vi "Subroutine Example.vi"() -> ()   [LabVIEW 2019]
uses:
  <vilib>/gpm_packages/@cs/test-executive/Source/Test Executive/TestExecutive/Test Executive.lvclass
  C:/Program Files/National Instruments/LabVIEW 2019/vi.lib/gpm_packages/@cs/test-executive/Source/Test Executive/ITestExecutive/ITest Executive.lvclass
  <vilib>/gpm_packages/@cs/persistence/source/XML/XML.lvclass
  C:/Program Files/National Instruments/LabVIEW 2019/vi.lib/gpm_packages/@cs/persistence/source/IPersist/IPersist.lvclass
  <vilib>/gpm_packages/@cs/test-executive/Source/Test Executive/Executioner/Executioner.lvclass
  <vilib>/gpm_packages/@cs/test-executive/Source/Test Executive/TestExecutive Ref/TestExecutive Ref.lvclass
  907dcd56-9374-434c-9b61-223c76acbea6.vi
  b311528a-8885-46dc-880b-1248f53f849d.vi
  <vilib>/gpm_packages/@cs/run-time-assertions/Source/Assert Equal/Assert Equal.lvclass
  cdae3e82-8768-4ad8-b607-63d253822acd.vi
  70d01af1-a21d-4a89-960c-204e12f52ec9.vi
  fcedef66-c37f-4fec-9b65-1c54ba2e8624.vi
  f2235a25-2eab-467c-a315-b32e95189d54.vi
  <vilib>/gpm_packages/@cs/test-executive/Source/Sandbox/While Loop Stop Example/Mock Executioner/Mock Executioner.lvclass
  65bccb3a-65fa-47ab-80ee-1967ce04f6c9.vi
  06bca68b-79a8-4024-9cd4-aed976a9ea7c.vi
  43d0685a-3af2-457a-b80b-c7e9f70f9eef.vi
  a6ff4ce3-d06d-4066-9c6d-186ba633a42e.vi
  C:/Program Files/National Instruments/LabVIEW 2019/vi.lib/gpm_packages/@cs/run-time-assertions/Source/Assert/Assert.lvclass
panel:
  out "Active Unique ID out":string
  out "Value":i32
  in  "Subroutine Test Exec":string(tree)
  in  "stop":bool
  in  "Saved Test Exec":string(tree)
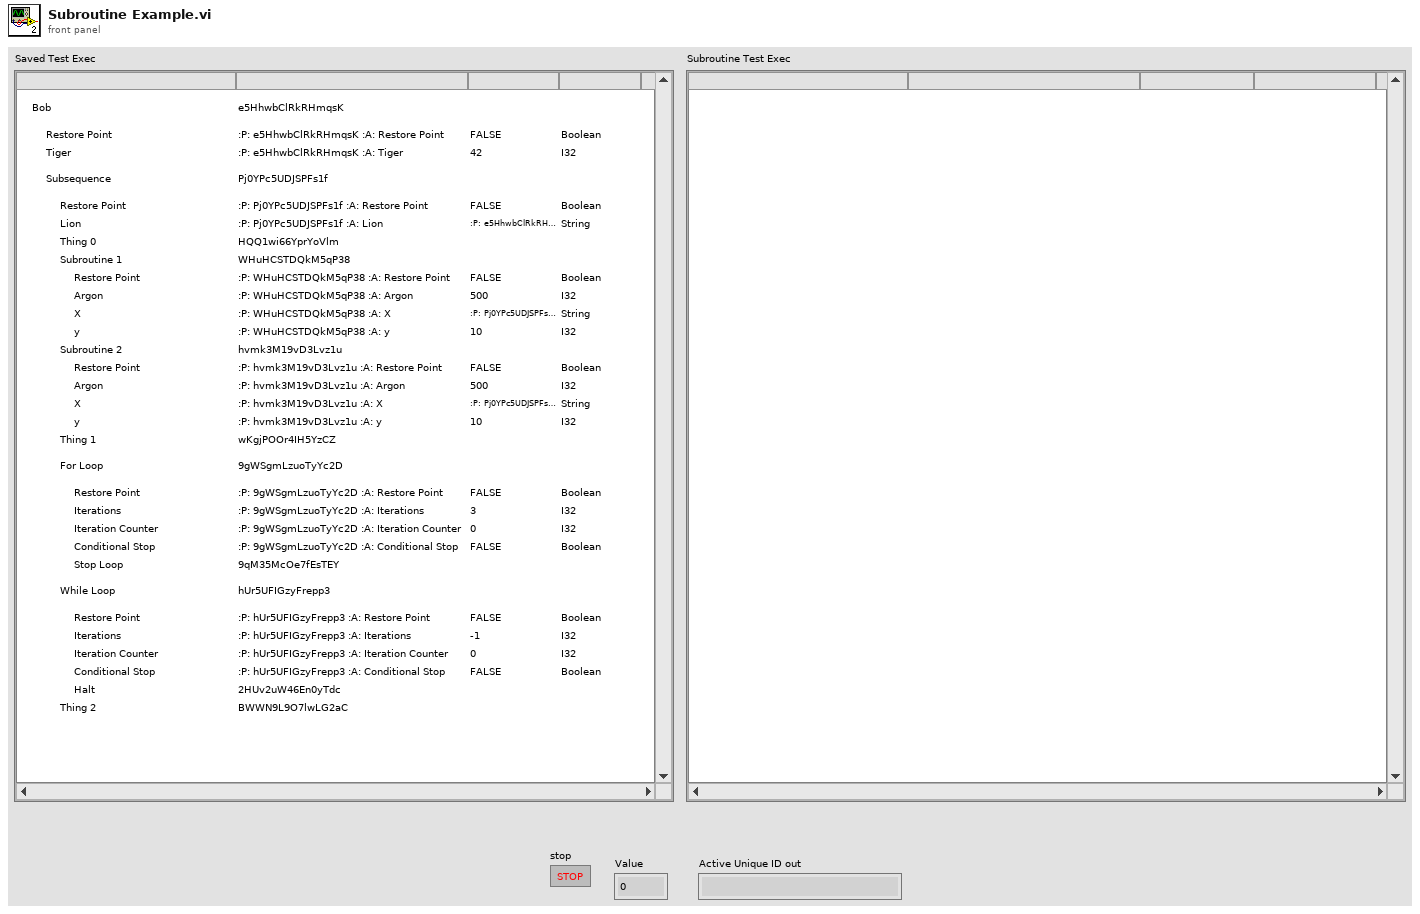
[diagram p1: front panel]
types:
  T1 = cluster{"Left Cell String":string, "Child Text":string[], "Child Tag":string, "Item Indent":i32, "Child Only?":bool, "Glyph Index":i32}[]
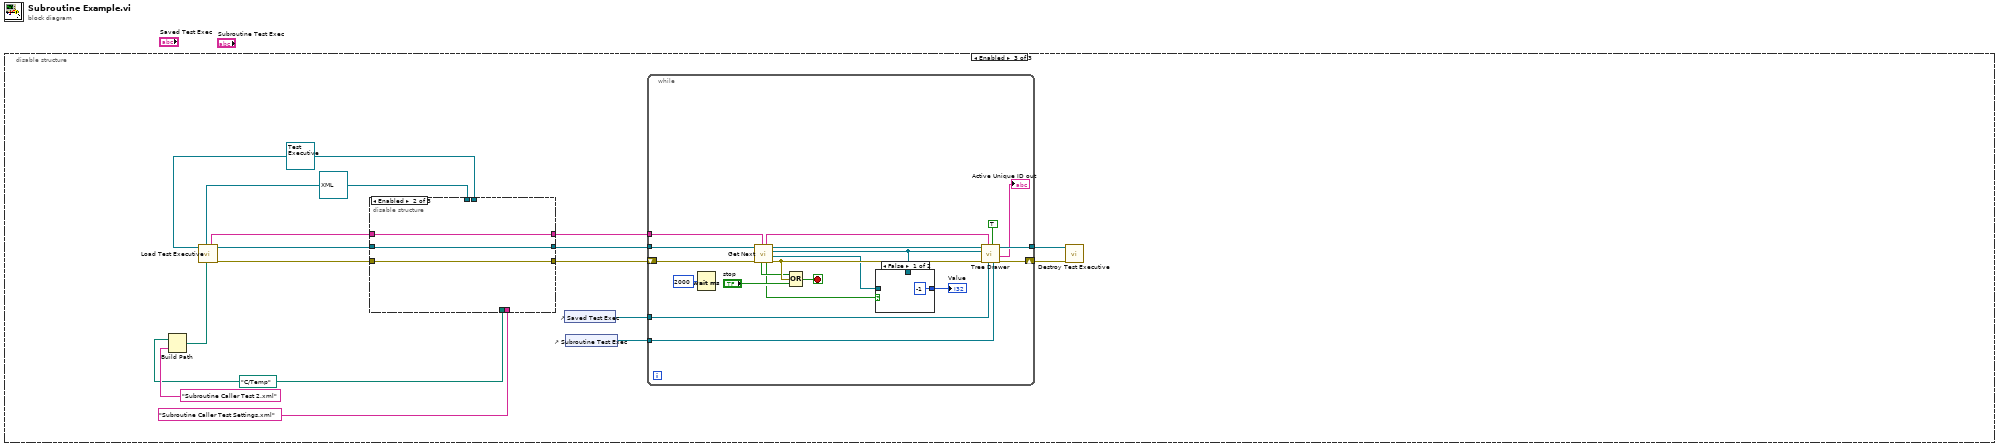
[diagram p0: block diagram]
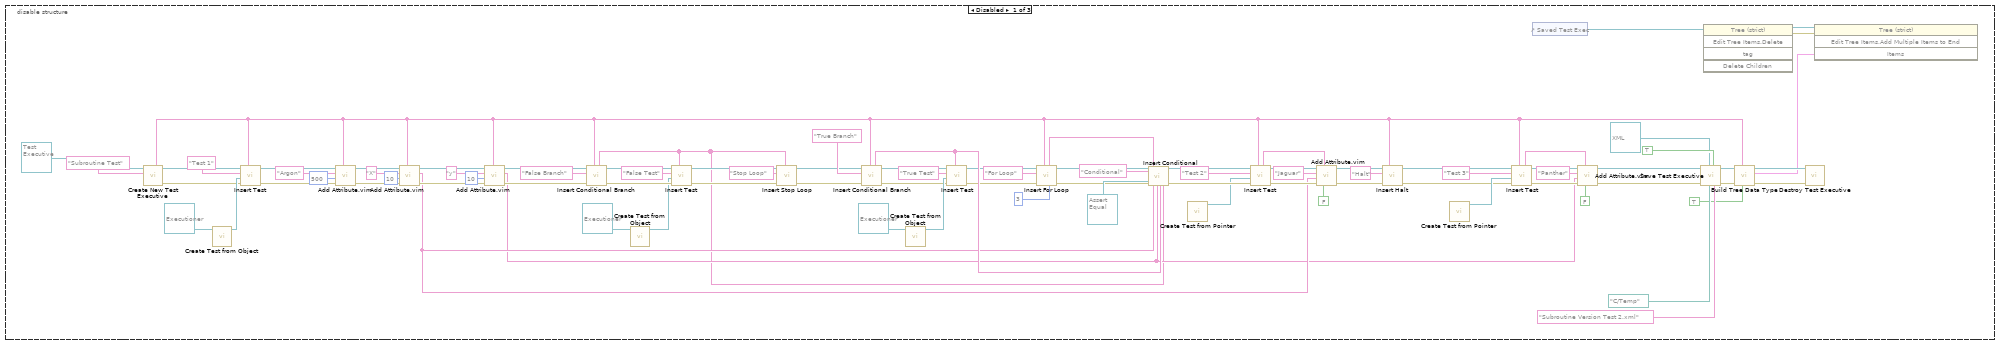
[diagram p2: hidden frame]
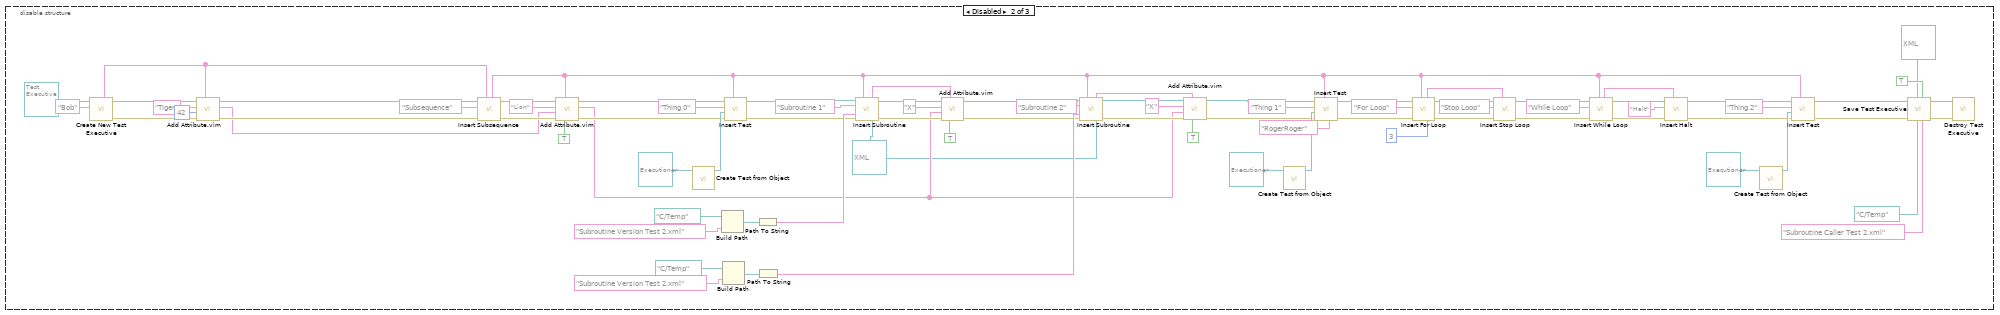
[diagram p3: hidden frame]
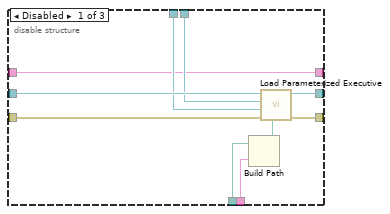
[diagram p4: hidden frame]
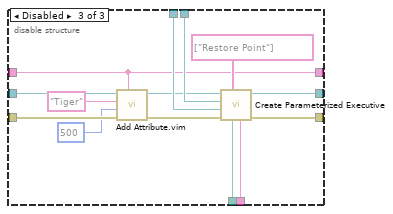
[diagram p5: hidden frame]
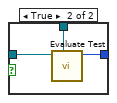
[diagram p6: hidden frame]
diagram:
  n1 = disable-structure shown="Enabled" {
    frame Disabled {
      n2 = call <vilib>:"Create New Test Executive.vi"("Name"="Subroutine Test", "Test Executive"=refnum<class "Test Executive.lvclass"> refnum ("Test Executive.lvlib:Test Executive.lvclass")) -> ("error out"=w82:errorcluster, "Test Executive Ref"=w83:refnum<data-value>, "Test Executive ID out"=w8:string)  [unwired: 7 in]
      n3 = call <vilib>:"Create Test from Object.vi"("Test"=refnum<class "Executioner.lvclass"> refnum ("Test Executive.lvlib:Executioner.lvclass")) -> ("Test"=w84:refnum<class "Executioner.lvclass">)  [unwired: 10 in]
      n4 = call <vilib>:"Insert Test.vi"("Parent ID"=w8, "error in (no error)"=w82, "Test"=w84, "Name"="Test 1", "Test Executive Ref"=w83) -> ("error out"=w34:errorcluster, "Test Executive Ref out"=w36:refnum<data-value>)  [unwired: 3 in, 2 out]
      n5 = call "Add Attribute.vim"("ID"=w8, "error in (no error)"=w34, "Attribute"=500, "Attribute Name"="Argon", "Test Executive Ref"=w36) -> ("error out"=w33:errorcluster, "Test Executive Ref out"=w35:refnum<data-value>)  [unwired: 3 in, 2 out]
      n6 = call "Add Attribute.vim"("ID"=w8, "error in (no error)"=w33, "Attribute"=10, "Attribute Name"="X", "Test Executive Ref"=w35) -> ("error out"=w74:errorcluster, "Attribute ID out"=w40:string, "Test Executive Ref out"=w75:refnum<data-value>)  [unwired: 3 in, 1 out]
      n7 = call "Add Attribute.vim"("ID"=w8, "error in (no error)"=w74, "Attribute"=10, "Attribute Name"="y", "Test Executive Ref"=w75) -> ("error out"=w68:errorcluster, "Attribute ID out"=w22:string, "Test Executive Ref out"=w69:refnum<data-value>)  [unwired: 3 in, 1 out]
      n8 = call <vilib>:"Insert Conditional Branch.vi"("Parent ID"=w8, "error in (no error)"=w68, "Name"="False Branch", "Test Executive Ref"=w69) -> ("error out"=w72:errorcluster, "Test Executive Ref out"=w71:refnum<data-value>, "Unique ID out"=w2:string)  [unwired: 4 in, 1 out]
      n9 = call <vilib>:"Create Test from Object.vi"("Test"=refnum<class "Executioner.lvclass"> refnum ("Test Executive.lvlib:Executioner.lvclass")) -> ("Test"=w66:refnum<class "Executioner.lvclass">)  [unwired: 10 in]
      n10 = call <vilib>:"Insert Test.vi"("Parent ID"=w2, "error in (no error)"=w72, "Test"=w66, "Name"="False Test", "Test Executive Ref"=w71) -> ("error out"=w4:errorcluster, "Test Executive Ref out"=w6:refnum<data-value>)  [unwired: 3 in, 2 out]
      n11 = call <vilib>:"Insert Stop Loop.vi"("Parent ID"=w2, "error in (no error)"=w4, "Name"="Stop Loop", "Test Executive Ref"=w6) -> ("error out"=w3:errorcluster, "Test Executive Ref out"=w5:refnum<data-value>)  [unwired: 4 in, 2 out]
      n12 = call <vilib>:"Insert Conditional Branch.vi"("Parent ID"=w8, "error in (no error)"=w3, "Name"="True Branch", "Test Executive Ref"=w5) -> ("error out"=w62:errorcluster, "Test Executive Ref out"=w63:refnum<data-value>, "Unique ID out"=w58:string)  [unwired: 4 in, 1 out]
      n13 = call <vilib>:"Create Test from Object.vi"("Test"=refnum<class "Executioner.lvclass"> refnum ("Test Executive.lvlib:Executioner.lvclass")) -> ("Test"=w65:refnum<class "Executioner.lvclass">)  [unwired: 10 in]
      n14 = call <vilib>:"Insert Test.vi"("Parent ID"=w58, "error in (no error)"=w62, "Test"=w65, "Name"="True Test", "Test Executive Ref"=w63) -> ("error out"=w10:errorcluster, "Test Executive Ref out"=w12:refnum<data-value>)  [unwired: 3 in, 2 out]
      n15 = call <vilib>:"Insert For Loop.vi"("Loop Iterations"=3, "Parent ID"=w8, "error in (no error)"=w10, "Name"="For Loop", "Test Executive Ref"=w12) -> ("error out"=w9:errorcluster, "Test Executive Ref out"=w11:refnum<data-value>, "Unique ID out"=w7:string)  [unwired: 3 in, 1 out]
      n16 = call <vilib>:"Insert Conditional.vi"("Test Executive Ref"=w11, "Name"="Conditional", "Assertion"=refnum<class "Assert Equal.lvclass"> refnum ("Run Time Assertions.lvlib:Assert Equal.lvclass"), "error in (no error)"=w9, "Parent ID"=w7, "Variable X"=w40, "Variable Y"=w22, "Passing Executive"=w58, "Failing Executive"=w2) -> ("Test Executive Ref out"=w56:refnum<data-value>, "error out"=w55:errorcluster)  [unwired: 7 in, 2 out]
      n17 = call <vilib>:"Create Test from Pointer.vi"() -> ("Test"=w39:refnum<class "Executioner.lvclass">)  [unwired: 11 in]
      n18 = call <vilib>:"Insert Test.vi"("Parent ID"=w8, "error in (no error)"=w55, "Test"=w39, "Name"="Test 2", "Test Executive Ref"=w56) -> ("error out"=w44:errorcluster, "Test Executive Ref out"=w45:refnum<data-value>, "Unique ID out"=w43:string)  [unwired: 3 in, 1 out]
      n19 = call "Add Attribute.vim"("Pointer?"=FALSE, "ID"=w43, "error in (no error)"=w44, "Attribute"=w40, "Attribute Name"="Jaguar", "Test Executive Ref"=w45) -> ("error out"=w18:errorcluster, "Test Executive Ref out"=w21:refnum<data-value>)  [unwired: 2 in, 2 out]
      n20 = call <vilib>:"Insert Halt.vi"("Parent ID"=w8, "error in (no error)"=w18, "Name"="Halt", "Test Executive Ref"=w21) -> ("error out"=w17:errorcluster, "Test Executive Ref out"=w20:refnum<data-value>)  [unwired: 4 in, 2 out]
      n21 = call <vilib>:"Create Test from Pointer.vi"() -> ("Test"=w31:refnum<class "Executioner.lvclass">)  [unwired: 11 in]
      n22 = call <vilib>:"Insert Test.vi"("Parent ID"=w8, "error in (no error)"=w17, "Test"=w31, "Name"="Test 3", "Test Executive Ref"=w20) -> ("error out"=w27:errorcluster, "Test Executive Ref out"=w26:refnum<data-value>, "Unique ID out"=w28:string)  [unwired: 3 in, 1 out]
      n23 = control-ref of="Saved Test Exec"() -> (w47:refnum<vi>)
      n24 = call "Add Attribute.vim"("Pointer?"=FALSE, "ID"=w28, "error in (no error)"=w27, "Attribute"=w22, "Attribute Name"="Panther", "Test Executive Ref"=w26) -> ("error out"=w24:errorcluster, "Test Executive Ref out"=w23:refnum<data-value>)  [unwired: 2 in, 2 out]
      n25 = call <vilib>:"Save Test Executive.vi"("File Name"="Subroutine Version Test 2.xml", "New GUIDs"=TRUE, "Folder"=path "C:/Temp", "Persistence in"=refnum<class "XML.lvclass"> refnum ("XML.lvlib:XML.lvclass"), "error in (no error)"=w24, "Test Executive Ref"=w23) -> ("error out"=w53:errorcluster, "Test Executive Ref out"=w51:refnum<data-value>)  [unwired: 4 in]
      n26 = invoke on="Invoke Node" class="Tree (strict)" method="Edit Tree Items.Delete"(reference=w47) -> (reference out=w48:refnum<vi>, error out=w49:errorcluster)  [unwired: 4 in, 3 out]
      n27 = call <vilib>:"Build Tree Data Type.vi"("Show IDs (True)"=TRUE, "Test ID"=w8, "error in (no error)"=w53, "Test Executive Ref"=w51) -> ("error out"=w52:errorcluster, "Tree Data"=w46:T1, "Test Executive Ref out"=w50:refnum<data-value>)  [unwired: 5 in]
      n28 = call <vilib>:"Destroy Test Executive.vi"("error in (no error)"=w52, "Test Executive Ref"=w50) -> ()  [unwired: 9 in, 1 out]
      n29 = invoke on="Invoke Node" class="Tree (strict)" method="Edit Tree Items.Add Multiple Items to End"(reference=w48, error in=w49, "Items"=w46) -> ()  [unwired: 1 in, 4 out]
    }
    frame Disabled {
      w90 = refnum<class "XML.lvclass"> refnum ("XML.lvlib:XML.lvclass")
      n30 = call <vilib>:"Create New Test Executive.vi"("Name"="Bob", "Test Executive"=refnum<class "Test Executive.lvclass"> refnum ("Test Executive.lvlib:Test Executive.lvclass")) -> ("error out"=w134:errorcluster, "Test Executive Ref"=w136:refnum<data-value>, "Test Executive ID out"=w132:string)  [unwired: 7 in]
      n31 = call "Add Attribute.vim"("ID"=w132, "error in (no error)"=w134, "Attribute"=42, "Attribute Name"="Tiger", "Test Executive Ref"=w136) -> ("error out"=w133:errorcluster, "Attribute ID out"=w125:string, "Test Executive Ref out"=w135:refnum<data-value>)  [unwired: 3 in, 1 out]
      n32 = call <vilib>:"Insert Subsequence.vi"("Parent ID"=w132, "error in (no error)"=w133, "Name"="Subsequence", "Test Executive Ref"=w135) -> ("error out"=w129:errorcluster, "Test Executive Ref out"=w131:refnum<data-value>, "Unique ID out"=w98:string)  [unwired: 4 in, 1 out]
      n33 = call "Add Attribute.vim"("Pointer?"=TRUE, "ID"=w98, "error in (no error)"=w129, "Attribute"=w125, "Attribute Name"="Lion", "Test Executive Ref"=w131) -> ("error out"=w128:errorcluster, "Attribute ID out"=w110:string, "Test Executive Ref out"=w130:refnum<data-value>)  [unwired: 2 in, 1 out]
      n34 = call <vilib>:"Create Test from Object.vi"("Test"=refnum<class "Executioner.lvclass"> refnum ("Test Executive.lvlib:Executioner.lvclass")) -> ("Test"=w143:refnum<class "Executioner.lvclass">)  [unwired: 10 in]
      n35 = Build Path(base path=path "C:/Temp" ("Folder"), name or relative path="Subroutine Version Test 2.xml" ("File Name")) -> (appended path=w159:path)
      n36 = Build Path(base path=path "C:/Temp" ("Folder"), name or relative path="Subroutine Version Test 2.xml" ("File Name")) -> (appended path=w154:path)
      n37 = call <vilib>:"Insert Test.vi"("Parent ID"=w98, "error in (no error)"=w128, "Test"=w143, "Name"="Thing 0", "Test Executive Ref"=w130) -> ("error out"=w139:errorcluster, "Test Executive Ref out"=w140:refnum<data-value>)  [unwired: 3 in, 2 out]
      n38 = Path To String(path=w159) -> (string=w145:string)
      n39 = Path To String(path=w154) -> (string=w144:string)
      n40 = call <vilib>:"Insert Subroutine.vi"("Test Executive Ref"=w140, "Parent ID"=w98, "Name"="Subroutine 1", "Subroutine Path"=w145, "error in (no error)"=w139, "Persistence"=w90) -> ("Unique ID out"=w119:string, "Test Executive Ref out"=w123:refnum<data-value>, "error out"=w121:errorcluster)  [unwired: 6 in, 1 out]
      n41 = call "Add Attribute.vim"("Pointer?"=TRUE, "ID"=w119, "error in (no error)"=w121, "Attribute"=w110, "Attribute Name"="X", "Test Executive Ref"=w123) -> ("error out"=w120:errorcluster, "Test Executive Ref out"=w122:refnum<data-value>)  [unwired: 2 in, 2 out]
      n42 = call <vilib>:"Insert Subroutine.vi"("Test Executive Ref"=w122, "Parent ID"=w98, "Name"="Subroutine 2", "Subroutine Path"=w144, "error in (no error)"=w120, "Persistence"=w90) -> ("Unique ID out"=w111:string, "Test Executive Ref out"=w115:refnum<data-value>, "error out"=w113:errorcluster)  [unwired: 6 in, 1 out]
      n43 = call "Add Attribute.vim"("Pointer?"=TRUE, "ID"=w111, "error in (no error)"=w113, "Attribute"=w110, "Attribute Name"="X", "Test Executive Ref"=w115) -> ("error out"=w112:errorcluster, "Test Executive Ref out"=w114:refnum<data-value>)  [unwired: 2 in, 2 out]
      n44 = call <vilib>:"Create Test from Object.vi"("Test"=refnum<class "Executioner.lvclass"> refnum ("Test Executive.lvlib:Executioner.lvclass")) -> ("Test"=w165:refnum<class "Executioner.lvclass">)  [unwired: 10 in]
      n45 = call <vilib>:"Insert Test.vi"("Unique ID"="RogerRoger", "Parent ID"=w98, "error in (no error)"=w112, "Test"=w165, "Name"="Thing 1", "Test Executive Ref"=w114) -> ("error out"=w106:errorcluster, "Test Executive Ref out"=w107:refnum<data-value>)  [unwired: 2 in, 2 out]
      n46 = call <vilib>:"Insert For Loop.vi"("Loop Iterations"=3, "Parent ID"=w98, "error in (no error)"=w106, "Name"="For Loop", "Test Executive Ref"=w107) -> ("error out"=w102:errorcluster, "Test Executive Ref out"=w103:refnum<data-value>, "Unique ID out"=w101:string)  [unwired: 3 in, 1 out]
      n47 = call <vilib>:"Insert Stop Loop.vi"("Parent ID"=w101, "error in (no error)"=w102, "Name"="Stop Loop", "Test Executive Ref"=w103) -> ("error out"=w97:errorcluster, "Test Executive Ref out"=w99:refnum<data-value>)  [unwired: 4 in, 2 out]
      n48 = call <vilib>:"Insert While Loop.vi"("Parent ID"=w98, "error in (no error)"=w97, "Name"="While Loop", "Test Executive Ref"=w99) -> ("error out"=w94:errorcluster, "Test Executive Ref out"=w95:refnum<data-value>, "Unique ID out"=w93:string)  [unwired: 4 in, 1 out]
      n49 = call <vilib>:"Insert Halt.vi"("Parent ID"=w93, "error in (no error)"=w94, "Name"="Halt", "Test Executive Ref"=w95) -> ("error out"=w91:errorcluster, "Test Executive Ref out"=w92:refnum<data-value>)  [unwired: 4 in, 2 out]
      n50 = call <vilib>:"Create Test from Object.vi"("Test"=refnum<class "Executioner.lvclass"> refnum ("Test Executive.lvlib:Executioner.lvclass")) -> ("Test"=w164:refnum<class "Executioner.lvclass">)  [unwired: 10 in]
      n51 = call <vilib>:"Insert Test.vi"("Parent ID"=w98, "error in (no error)"=w91, "Test"=w164, "Name"="Thing 2", "Test Executive Ref"=w92) -> ("error out"=w155:errorcluster, "Test Executive Ref out"=w156:refnum<data-value>)  [unwired: 3 in, 2 out]
      n52 = call <vilib>:"Save Test Executive.vi"("File Name"="Subroutine Caller Test 2.xml", "New GUIDs"=TRUE, "Folder"=path "C:/Temp", "Persistence in"=refnum<class "XML.lvclass"> refnum ("XML.lvlib:XML.lvclass"), "error in (no error)"=w155, "Test Executive Ref"=w156) -> ("error out"=w150:errorcluster, "Test Executive Ref out"=w151:refnum<data-value>)  [unwired: 4 in]
      n53 = call <vilib>:"Destroy Test Executive.vi"("error in (no error)"=w150, "Test Executive Ref"=w151) -> ()  [unwired: 9 in, 1 out]
    }
    frame Enabled {
      w174 = refnum<class "XML.lvclass"> refnum ("XML.lvlib:XML.lvclass")
      w175 = refnum<class "Test Executive.lvclass"> refnum ("Test Executive.lvlib:Test Executive.lvclass")
      w173 = path "C:/Temp" ("Folder")
      n54 = Build Path(base path=w173, name or relative path="Subroutine Caller Test 2.xml" ("File Name")) -> (appended path=w181:path)
      n55 = call <vilib>:"Load Test Executive.vi"("Folder"=w181, "Persistence in"=w174, "Test Executive"=w175) -> ("error out"=w177:errorcluster, "Test Executive Ref out"=w179:refnum<data-value>, "Root ID"=w171:string)  [unwired: 6 in]
      n56 = disable-structure shown="Enabled" {
        disable-tunnel: w179 -> [w195 w197 w205]
        disable-tunnel: [w194 w197 w212] -> w178
        disable-tunnel: w177 -> [w193 w196 w203]
        disable-tunnel: [w192 w196 w211] -> w176
        disable-tunnel: w175 -> [w191 _ w208]
        disable-tunnel: w174 -> [w190 _ w207]
        disable-tunnel: w173 -> [w189 _ w210]
        disable-tunnel: "Subroutine Caller Test Settings.xml" ("File Name") -> [w188 _ w209]
        disable-tunnel: [w186 w198 w201] -> w170
        disable-tunnel: w171 -> [w186 w198 w201]
        frame Disabled {
          n57 = Build Path(base path=w189, name or relative path=w188) -> (appended path=w187:path)
          n58 = call <vilib>:"Load Parameterized Executive.vi"("Folder"=w187, "error in (no error)"=w193, "Persistence in"=w190, "Test Executive"=w191, "Test Executive Ref"=w195) -> ("error out"=w192:errorcluster, "Test Executive Ref out"=w194:refnum<data-value>)  [unwired: 5 in]
        }
        frame Enabled {
        }
        frame Disabled {
          n59 = call "Add Attribute.vim"("ID"=w201, "error in (no error)"=w203, "Attribute"=500, "Attribute Name"="Tiger", "Test Executive Ref"=w205) -> ("error out"=w202:errorcluster, "Test Executive Ref out"=w204:refnum<data-value>)  [unwired: 3 in, 2 out]
          n60 = call <vilib>:"Create Parameterized Executive.vi"("File Name"=w209, "Folder"=w210, "Attribute Name Blacklist"=string[] ["Restore Point"], "error in (no error)"=w202, "Persistence in"=w207, "Test Executive"=w208, "Test Executive Ref"=w204) -> ("error out"=w211:errorcluster, "Test Executive Ref out"=w212:refnum<data-value>)  [unwired: 3 in]
        }
      }
      n61 = control-ref of="Saved Test Exec"() -> (w183:refnum<vi>)
      n62 = control-ref of="Subroutine Test Exec"() -> (w180:refnum<vi>)
      n63 = while {
        shift-right: [w223] -> w184
        shift-left: w176 -> [w227]
        tunnel: w170 -> [w229]
        tunnel: w183 -> [w222]
        tunnel: w178 -> [w228]
        tunnel: [w225] -> w185
        tunnel: w180 -> [w221]
        stop <- w231 stop-if-true
        n64 = Wait (ms)(milliseconds to wait=u32 2000) -> ()  [unwired: 1 out]
        n65 = call <vilib>:"Get Next.vi"("Unique ID"=w229, "error in (no error)"=w227, "Test Executive Ref"=w228) -> ("error out"=w224:errorcluster, "Test"=w218:refnum<class "Executioner.lvclass">, "Active Test Executive Ref out"=w217:refnum<data-value>, "Test Executive Ref out"=w226:refnum<data-value>, "Found"=w214:bool, "Unique ID out"=w219:string, "Complete"=w215:bool)  [unwired: 2 in]
        n66 = Compound Arithmetic op=OR(w215, w224, "stop") -> (w231:bool)
        n67 = case shown="False" w214 {
          tunnel: w218 -> [_ w236]
          tunnel: w217 -> [_ w235]
          tunnel: [-1 ("Value") w234] -> w216
          frame False {
          }
          frame True {
            n68 = call <vilib>:"Evaluate Test.vi"("Test Executive Ref out"=w235, "Executioner in"=w236) -> ("Value"=w234:i32)  [unwired: 9 in]
          }
        }
        "Value" <- w216
        n69 = call "Tree Drawer"("Subroutine Tree Ref"=w221, "Show IDs (True)"=TRUE, "Test Exec Tree Ref"=w222, "Active Unique ID"=w219, "error in (no error)"=w224, "Active Test Executive Ref"=w217, "Test Executive Ref"=w226) -> ("error out"=w223:errorcluster, "Active Unique ID out"=→"Active Unique ID out":string, "Test Executive Ref out"=w225:refnum<data-value>)  [unwired: 1 in, 1 out]
      }
      n70 = call <vilib>:"Destroy Test Executive.vi"("error in (no error)"=w184, "Test Executive Ref"=w185) -> ()  [unwired: 9 in, 1 out]
    }
  }
